vi "LCD Create Custom Char.vi"(8 "Error In":errorcluster, 9 "LCD Character":T1, 10 "Custom Char Number":u8, 11 "ChipKit Resource":T3={"COM Port"="", "Board Type"=enum."ChipKit uC32", "Connection Type"=enum."USB / Serial", "Baud Rate (115200)"=0, "Bytes Per Packet (15)"=15, "DI Port Num Pins"=0, "DO Port Num Pins"=0}) -> (0 "Error Out":errorcluster, 3 "ChipKit Resource":T3={"COM Port"="", "Board Type"=enum."ChipKit uC32", "Connection Type"=enum."USB / Serial", "Baud Rate (115200)"=0, "Bytes Per Packet (15)"=15, "DI Port Num Pins"=0, "DO Port Num Pins"=0})   [LabVIEW 2011, in "LabVIEW Interface for ChipKit.lvlib"]
doc: "Creates a custom character, which can be later printed on the LCD. This function supports 5x8 pixels. Note, after creating a new character the LCD must be reinitilized using the LCD Init VI. The custom character can be printed using the LCD Print Custom Char VI."
uses:
  LabVIEW Interface for ChipKit.lvlib
  Private/Type Defs/Chipkit Resource.ctl
  Private/Type Defs/Board Type.ctl
  Private/Type Defs/Connection Type.ctl
  Private/Type Defs/LCD Character.ctl
  Private/Type Defs/LCD Char Row.ctl
  Private/Type Defs/Command.ctl
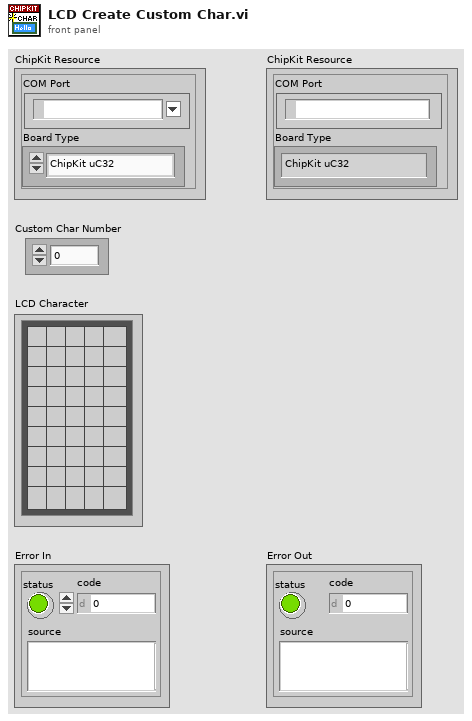
[diagram p1: front panel]
types:
  T1 = typedef "LabVIEW Interface for ChipKit.lvlib/LCD Character.ctl" = cluster{"Row 0":T2, "Row 1":T2, "Row 2":T2, "Row 3":T2, "Row 4":T2, "Row 5":T2, "Row 6":T2, "Row 7":T2, "Row 8":T2}
  T2 = typedef "LabVIEW Interface for ChipKit.lvlib/LCD Char Row.ctl" = cluster{"0":bool, "1":bool, "2":bool, "3":bool, "4":bool}
  T3 = typedef "LabVIEW Interface for ChipKit.lvlib/Chipkit Resource.ctl" = cluster{"COM Port":refnum<visa-resource-name>, "Board Type":T4, "Connection Type":T5, "Baud Rate (115200)":u32, "Bytes Per Packet (15)":u32, "DI Port Num Pins":i32, "DO Port Num Pins":i32}
  T4 = typedef "LabVIEW Interface for ChipKit.lvlib/Board Type.ctl" = enum16{"ChipKit uC32", "ChipKit Uno32", "ChipKit Max32"}
  T5 = typedef "LabVIEW Interface for ChipKit.lvlib/Connection Type.ctl" = enum8{"USB / Serial", "XBEE", "BlueSmirf (Bluetooth)"}
  T6 = typedef "LabVIEW Interface for ChipKit.lvlib/Command.ctl" = enum8{"setArduinoMode", "flushSerial", "setPinMode", "digitalWritePin", "digitalWritePort", "tone", "digitalReadPin", "digitalReadPort", "analogReadPin", "analogReadPort", "pwmWritePin", "pwmWritePort", "sevenSegment_Configure", "sevenSegment_Write", "I2C Init", "I2C Write", "I2C Read", "SPI Init", "SPI Set Bit Order", "SPI Set Clock Divider", "SPI Set Data Mode", "SPI Send / Receive", "SPI Close", "Servo Set Num Servos", "Servo Config Servo", "Servo Write Angle", "Servo Read Angle", "Servo Write Pulse Width", "Servo Read Pulse Width", "Servo Detach", "LCD Init", "LCD Set Size", "LCD Set Cursor Mode", "LCD Clear", "LCD Set Cursor Position", "LCD Print", "LCD Display Power", "LCD Scroll Display", "LCD Autoscroll", "LCD Print Direction", "LCD Create Custom Char", "LCD Print Custom Char", "contAcqOn", "contAcqOff", "getFirmwareVersion", "FiniteSampleStart", "NA", "NA2", "Conifg Stepper", "Stepper Write", "Stepper Detach", "Stepper Steps To Go", "Config DO Port", "Config DI Port"}
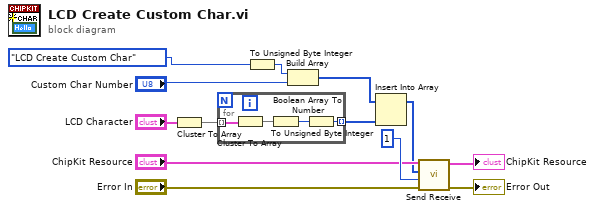
[diagram p0: block diagram]
diagram:
  n1 = Cluster To Array(cluster="LCD Character") -> (array=w5:T2[])
  n2 = for {
    tunnel: w5 -> [w17] mode=indexing
    tunnel: [w14] -> w4 mode=indexing
    n3 = Cluster To Array(cluster=w17) -> (array=w16:bool[])
    n4 = Boolean Array To Number(Boolean array=w16) -> (number=w15:u32)
    n5 = To Unsigned Byte Integer(number=w15) -> (unsigned 8bit integer=w14:u8)
  }
  n6 = To Unsigned Byte Integer(number=Command."LCD Create Custom Char" ("Command")) -> (unsigned 8bit integer=w12:u8)
  n7 = Build Array(w12, "Custom Char Number") -> (w3:u8[])
  n8 = Insert Into Array(array=w3, new element=w4) -> (w2:u8[])  [unwired: 1 in]
  n9 = call "Send Receive.vi"("Error In"="Error In", "Bytes To Read (0)"=u8 1, "Data"=w2, "ChipKit Resource"="ChipKit Resource") -> ("Error Out"=→"Error Out":errorcluster, "ChipKit Resource"=→"ChipKit Resource":T3)  [unwired: 5 in, 1 out]
